vi "Clapper set state.vi"(8 "error in":errorcluster, 9 "PotDevRef":T12={"DevStatus"={"status"=FALSE, "code"=0, "source"=""}, "Controller"=enum."Controller 1", "Analog Channel"=enum."AI 3", "Invert Output"=FALSE}, 10 "MotorControlDevRef":T3={"DeviceStatus"={"status"=FALSE, "code"=0, "source"=""}, "Type"=enum."CANTalonSRX", "PWM"={"Controller"=enum."Controller 1", "PWM Channel"=enum."PWM 1", "DeadBand"={"Name"="", "maxPositivePwm"=0, "minPositivePwm"=0, "centerPwm"=0, "maxNegativePwm"=0, "minNegativePwm"=0, "angularRange"=0}}, "CAN"={"Device Number"=1, "Control Mode"=enum."Percent VBus", "Semaphore"=refnum, "Max Vout"=12.0, "TalonSRX Control Mode"=enum."Percent VBus"}, "Invert"=FALSE, "TransformRef"=refnum, "InvTransformRef"=refnum}, 11 "Enum":T2) -> (0 "error out":errorcluster, 1 "Good enough?":bool)   [LabVIEW 2014]
uses:
  Arm clapper state.ctl
  <vilib>/Rock Robotics/WPI/Potentiometer/WPI_PotentiometerDevRef.ctl
  <vilib>/Rock Robotics/SystemInterfaces/Typedef/FPGA_TypedefAnalogModule.ctl
  <vilib>/Rock Robotics/SystemInterfaces/AI/FPGA_AIChannel.ctl
  <vilib>/Rock Robotics/WPI/MotorControl/WPI_MotorControlDeviceRef.ctl
  <vilib>/Rock Robotics/WPI/MotorControl/WPI_MotorControlType.ctl
  <vilib>/Rock Robotics/SystemInterfaces/Typedef/FPGA_TypedefDigitalModule.ctl
  <vilib>/Rock Robotics/SystemInterfaces/DIO/FPGA_DIOPWMChannel.ctl
  <vilib>/Rock Robotics/WPI/PWM/WPI_PWMDeadband.ctl
  <vilib>/Rock Robotics/WPI/CAN/Jaguar/SubVIs/WPI_CANJaguar_ControlMode.ctl
  <vilib>/Rock Robotics/WPI/CAN/TalonSRX/WPI_CANTalonSRX_APIControlMode.ctl
  <vilib>/Rock Robotics/WPI/PWM/WPI_PWMTransform_ConPane.ctl
  Clapper Control Mode.ctl
  <vilib>/Rock Robotics/WPI/DriverStation/WPI_DriverStationRobotMode2.ctl
  Robot Global Data.vi
  <vilib>/addons/control/pid/pid.llb/PID (DBL).vi
  <vilib>/Rock Robotics/Network Tables/SD Write Number.vi
  <vilib>/addons/control/pid/NI_PID_pid.lvlib
panel:
  in  "Tolerance":dbl=0.05 format="%#_13g"
  in  "Open":dbl=0.98 format="%#_13g"
  in  "In":dbl=0.36 format="%#_13g"
  in  "Tote Closed":dbl=0.658 format="%#_13g"
  in  "Bin Closed":dbl=0.701 format="%#_13g"
  in  "Straight":dbl=0.751 format="%#_13g"
  in  "Tab Control":T1(tab)=enum."Refs"
  in  "PID gains":T15={"proportional gain (Kc)"=2.0, "integral time (Ti, min)"=0.0, "derivative time (Td, min)"=0.0} {"proportional gain (Kc)" min=-10.0 max=10.0 step=0.0001; "integral time (Ti, min)" min=0.0 max=10.0 step=0.0001; "derivative time (Td, min)" min=0.0 max=10.0 step=0.0001}
  in  "output range":cluster{"output high":dbl, "output low":dbl}={"output high"=1.0, "output low"=-1.0}
  # "Controls"
  # "Indicators"
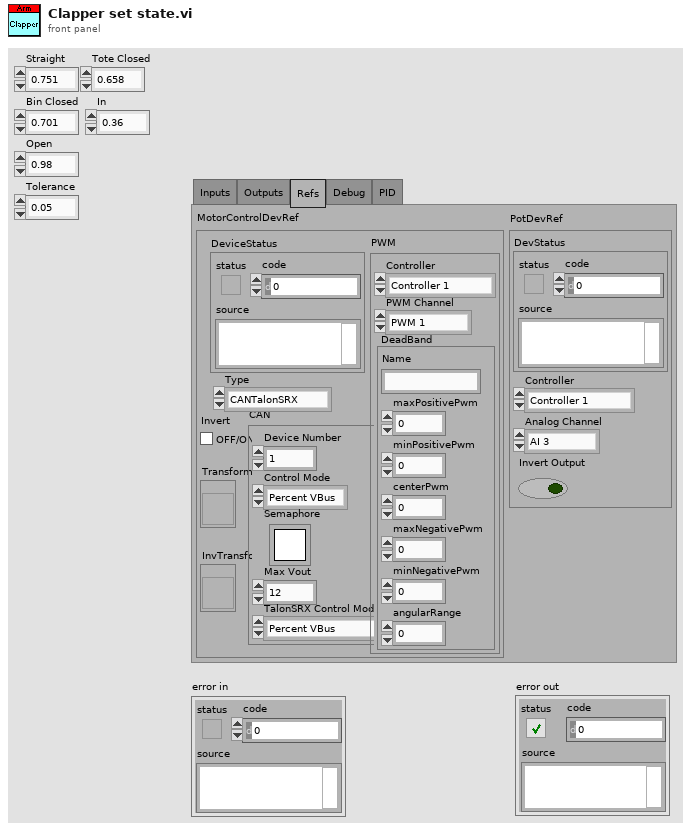
[diagram p1: front panel]
types:
  T1 = enum32{"Inputs", "Outputs", "Refs", "Debug", "PID"}
  T2 = typedef "Arm clapper state.ctl" = enum16{"In", "Tote Closed", "Bin Closed", "Straight", "Open"}
  T3 = typedef "WPI_MotorControlDeviceRef.ctl" = cluster{"DeviceStatus":errorcluster, "Type":T4, "PWM":cluster{"Controller":T5, "PWM Channel":T6, "DeadBand":T7}, "CAN":cluster{"Device Number":u8, "Control Mode":T8, "Semaphore":T9, "Max Vout":dbl, "TalonSRX Control Mode":T10}, "Invert":bool, "TransformRef":T11, "InvTransformRef":T11}
  T4 = typedef "WPI_MotorControlType.ctl" = enum16{"PWM", "CAN", "CANTalonSRX"}
  T5 = typedef "FPGA_TypedefDigitalModule.ctl" = enum16{"Controller 1"}
  T6 = typedef "FPGA_DIOPWMChannel.ctl" = enum8{"PWM 0", "PWM 1", "PWM 2", "PWM 3", "PWM 4", "PWM 5", "PWM 6", "PWM 7", "PWM 8", "PWM 9", "PWM MXP 0", "PWM MXP 1", "PWM MXP 2", "PWM MXP 3", "PWM MXP 4", "PWM MXP 5", "PWM MXP 6", "PWM MXP 7", "PWM MXP 8", "PWM MXP 9", "Invalid"}
  T7 = typedef "WPI_PWMDeadband.ctl" = cluster{"Name":string, "maxPositivePwm":i32, "minPositivePwm":i32, "centerPwm":i32, "maxNegativePwm":i32, "minNegativePwm":i32, "angularRange":u16}
  T8 = typedef "WPI_CANJaguar_ControlMode.ctl" = enum8{"Percent VBus", "Current", "Speed", "Position", "Voltage"}
  T9 = typedef "Semaphore RefNum" = refnum<k1>
  T10 = typedef "WPI_CANTalonSRX_APIControlMode.ctl" = enum8{"Percent VBus", "Speed", "Position", "Slave", "Unchanged / Invalid"}
  T11 = typedef "WPI_PWMTransform_ConPane.ctl" = refnum<vi>
  T12 = typedef "WPI_PotentiometerDevRef.ctl" = cluster{"DevStatus":errorcluster, "Controller":T13, "Analog Channel":T14, "Invert Output":bool}
  T13 = typedef "FPGA_TypedefAnalogModule.ctl" = enum16{"Controller 1"}
  T14 = typedef "FPGA_AIChannel.ctl" = enum8{"AI 0", "AI 1", "AI 2", "AI 3", "AI MXP 0", "AI MXP 1", "AI MXP 2", "AI MXP 3", "Invalid"}
  T15 = cluster{"proportional gain (Kc)":dbl, "integral time (Ti, min)":dbl, "derivative time (Td, min)":dbl}
  T16 = typedef "Clapper Control Mode.ctl" = enum16{"PID", "Manual"}
  T17 = typedef "WPI_DriverStationRobotMode2.ctl" = enum16{"Autonomous Disabled", "Autonomous Enabled", "Teleop Disabled", "Teleop Enabled", "Disconnected", "Finish", "Test Disabled", "Test Enabled", "Emergency Stopped"}
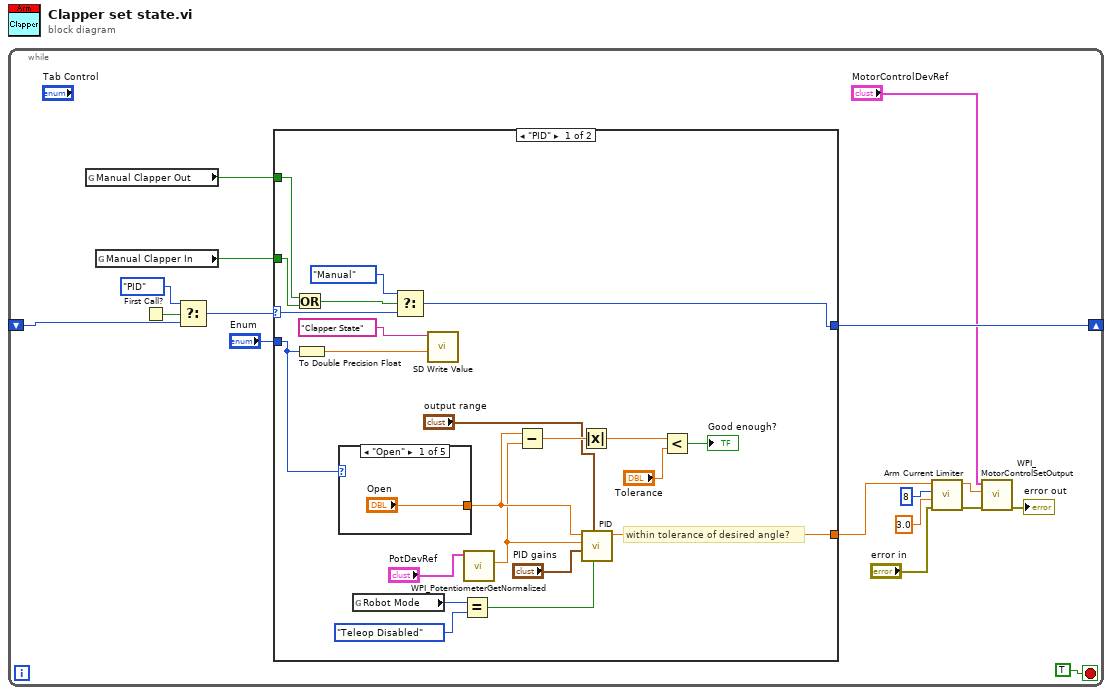
[diagram p0: block diagram]
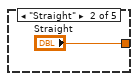
[diagram p2: hidden frame]
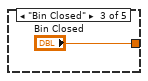
[diagram p3: hidden frame]
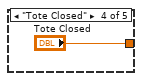
[diagram p4: hidden frame]
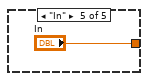
[diagram p5: hidden frame]
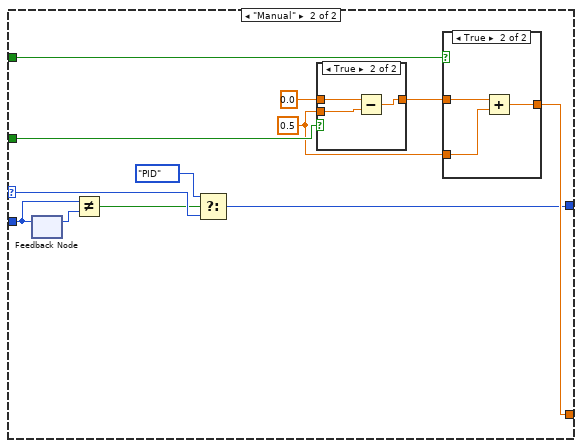
[diagram p6: hidden frame]
diagram:
  n1 = while {
    shift-right: [w15] -> _
    shift-left: _ -> [w12]
    stop <- TRUE stop-if-true
    n2 = global read "Robot Global Data.vi" "Manual Clapper Out"() -> (w9:bool)
    n3 = global read "Robot Global Data.vi" "Manual Clapper In"() -> (w16:bool)
    n4 = First Call?() -> (First Call?: T/F=w10:bool)
    n5 = Select(t=Clapper_Control_Mode."PID", s=w10, f=w12) -> (s? t:f=w13:T16)
    n6 = case shown="\"PID\"" w13 {
      selector: w13 -> [w35 w54]
      tunnel: [w27 w49] -> w8
      tunnel: "Enum" -> [w33 w53]
      tunnel: [w38 w48] -> w15
      tunnel: w9 -> [w36 w55]
      tunnel: w16 -> [w39 w56]
      frame "PID" {
        # "within tolerance of desired angle?"
        n7 = Or(x=w36, y=w39) -> (x .or. y?=w37:bool)
        n8 = To Double Precision Float(number=w33) -> (double precision float=w32:dbl)
        n9 = case shown="\"Open\"" w33 {
          tunnel: ["Open" "Straight" "Bin Closed" "Tote Closed" "In"] -> w29
          frame "Open" {
          }
          frame "Straight" {
          }
          frame "Bin Closed" {
          }
          frame "Tote Closed" {
          }
          frame "In" {
          }
        }
        n10 = global read "Robot Global Data.vi" "Robot Mode"() -> (w25:T17)
        n11 = Select(t=Clapper_Control_Mode."Manual", s=w37, f=w35) -> (s? t:f=w38:T16)
        n12 = call-poly <vilib>:"SD Write Value.vi"("Numeric"=w32, "Name"="Clapper State") -> ()  [unwired: 8 in, 2 out]
        n13 = Equal?(x=w25, y=WPI_DriverStationRobotMode2."Teleop Disabled") -> (x = y?=w26:bool)
        n14 = call <vilib>:"WPI_PotentiometerGetNormalized.vi"("PotDevRef"="PotDevRef") -> ("Normalized Value"=w18:dbl)  [unwired: 8 in, 2 out]
        n15 = Subtract(x=w29, y=w18) -> (x-y=w30:dbl)
        n16 = Absolute Value(x=w30) -> (abs(x)=w21:dbl)
        n17 = call-poly <vilib>:"PID.vi"("reinitialize? (F)"=w26, "output range"="output range", "PID gains"="PID gains", "process variable"=w18, "setpoint"=w29) -> ("output"=w27:dbl)  [unwired: 5 in, 1 out]
        n18 = Less?(x=w21, y="Tolerance") -> (x < y?=→"Good enough?":bool)
      }
      frame "Manual" {
        w50 = 0.5
        n19 = feedback #1() -> (w46:T2)  [unwired: 1 in]
        n20 = feedback-in #1(w53) -> ()
        n21 = Not Equal?(x=w53, y=w46) -> (x != y?=w47:bool)
        n22 = Select(t=Clapper_Control_Mode."PID", s=w47, f=w54) -> (s? t:f=w48:T16)
        n23 = case shown="True" w56 {
          tunnel: 0.0 -> [w57 w60]
          tunnel: w50 -> [_ w59]
          tunnel: [w57 w58] -> w52
          frame False {
          }
          frame True {
            n24 = Subtract(x=w60, y=w59) -> (x-y=w58:dbl)
          }
        }
        n25 = case shown="True" w55 {
          tunnel: w52 -> [w61 w64]
          tunnel: [w61 w62] -> w49
          tunnel: w50 -> [_ w63]
          frame False {
          }
          frame True {
            n26 = Add(x=w64, y=w63) -> (x+y=w62:dbl)
          }
        }
      }
    }
    n27 = call "Arm Current Limiter.vi"("Motor Input"=w8, "PDP Channel for arm motor"=8, "Max Current"=3.0, "error in"="error in") -> ("Set Motor To"=w7:dbl, "error out"=w6:errorcluster)  [unwired: 5 in]
    n28 = call <vilib>:"WPI_MotorControlSetOutput.vi"("error in (no error)"=w6, "Output"=w7, "MotorControlDevRef"="MotorControlDevRef") -> ("error out"=→"error out":errorcluster)  [unwired: 6 in, 2 out]
  }
